vi "Compile And Deploy.vi"(11 "target in":refnum<class "FPGATarget.lvclass">) -> (3 "target out":refnum<class "FPGATarget.lvclass">)   [LabVIEW 2020, in "NI_TargetHelper.lvlib" / "FPGATarget.lvclass"]
uses:
  <vilib>/TargetSupport/NI_TargetHelper/FPGATarget/FPGATarget.lvclass
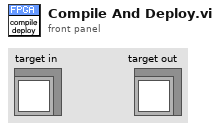
[diagram p1: front panel]
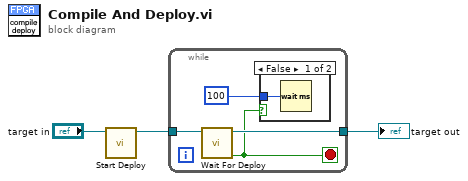
[diagram p0: block diagram]
diagram:
  n1 = call-dynamic "Start Deploy.vi"("FPGAtarget in"="target in") -> ("FPGAtarget out"=w1:refnum<class "FPGATarget.lvclass">)  [unwired: 10 in]
  n2 = while {
    tunnel: w1 -> [w7]
    tunnel: [w6] -> w2
    stop <- w5 stop-if-true
    n3 = call-dynamic "Wait For Deploy.vi"("FPGAtarget in"=w7) -> ("deployed"=w5:bool, "FPGAtarget out"=w6:refnum<class "FPGATarget.lvclass">)  [unwired: 9 in]
    n4 = case shown="False" w5 {
      tunnel: u32 100 -> [w8 _]
      frame False {
        n5 = Wait (ms)(milliseconds to wait=w8) -> ()  [unwired: 1 out]
      }
      frame True {
      }
    }
  }
  "target out" <- w2
